vi "update.links.request.vi"(8 "error in":errorcluster, 11 "Links":map{string, string}(c390)) -> (0 "error out":errorcluster, 1 "Request":string)   [LabVIEW 2020, in "Run.lvclass"]
uses:
  Run.lvclass
  e085151d-f813-46c9-b9d0-95cd78f8561e.vi
  <vilib>/JDP Science/JSONtext/Variant to JSON Text.vi
  <vilib>/JDP Science/JSONtext/support/Format JSON Array Text.vi
  <vilib>/JDP Science/JSONtext/support/Format JSON Object.vi
  <vilib>/JDP Science/JSONtext/LVClass Serializer/JSONtext LVClass Serializer.lvclass
  <vilib>/JDP Science/JSONtext/JSONtext.lvlib
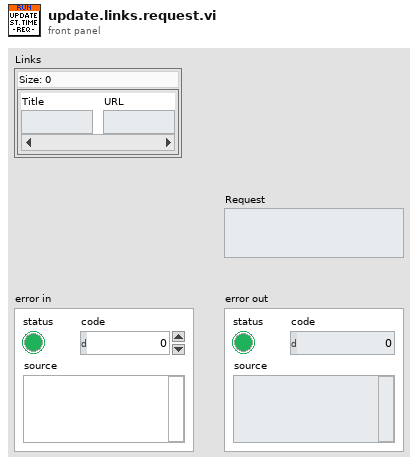
[diagram p1: front panel]
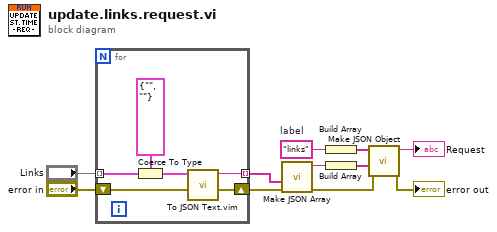
[diagram p0: block diagram]
diagram:
  w7 = "links"  # label
  n1 = for {
    tunnel: "Links" -> [w17] mode=indexing
    tunnel: [w16] -> w9 mode=indexing
    shift-right: [w15] -> w3
    shift-left: "error in" -> [w14]
    n2 = Coerce To Type(0:w17, 1:cluster{"url":string, "title":string} {"url"="", "title"=""} ("type")) -> (2:w13:cluster{"url":string, "title":string})
    n3 = call "To JSON Text.vim"("error in (no error)"=w14, "Anything"=w13) -> ("error out"=w15:errorcluster, "<JSON>"=w16:string)  [unwired: 8 in]
  }
  n4 = call <vilib>:"Make JSON Array.vi"("error in (no error)"=w3, "JSON Elements"=w9) -> ("error out"=w2:errorcluster, "<JSON>"=w5:string)  [unwired: 8 in]
  n5 = Build Array(w7) -> (w8:string[])
  n6 = Build Array(w5) -> (w6:string[])
  n7 = call <vilib>:"Make JSON Object.vi"("error in (no error)"=w2, "JSON Items"=w6, "Item Names"=w8) -> ("error out"=→"error out":errorcluster, "<JSON>"=→"Request":string)  [unwired: 7 in]
